vi "DestroyCommunication.vi"(8 "error in (no error)":errorcluster, 11 "Message Queues":T1) -> (0 "error out":errorcluster)   [LabVIEW 2017, in "Client.lvlib" / "CommsFrameWork.lvlib"]
doc: "Destroys all Queues and User Events."
uses:
  CommsFrameWork.lvlib
  TypeDefs/CommReferences.ctl
  ServerLib/SubLibs/Message Queue/MessageCluster.ctl
  ServerLib/SubLibs/Message Queue/Message Queue.lvlib
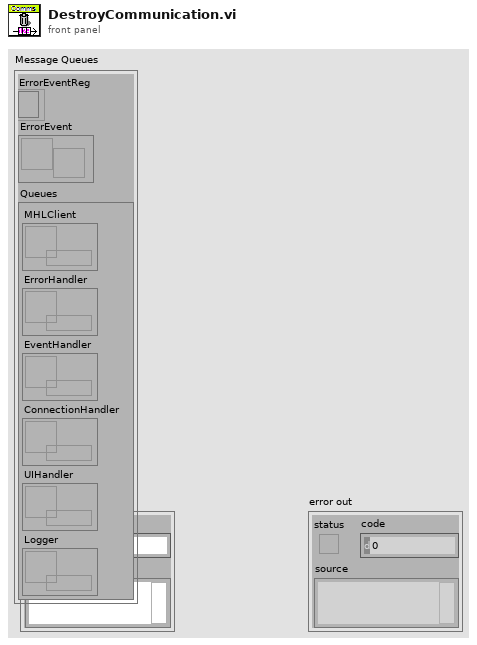
[diagram p1: front panel]
types:
  T1 = typedef "Client.lvlib/CommsFrameWork.lvlib/CommReferences.ctl" = cluster{"ErrorEventReg":refnum<event-registration>, "ErrorEvent":refnum<user-event>, "Queues":cluster{"MHLClient":refnum<queue>, "ErrorHandler":refnum<queue>, "EventHandler":refnum<queue>, "ConnectionHandler":refnum<queue>, "UIHandler":refnum<queue>, "Logger":refnum<queue>}}
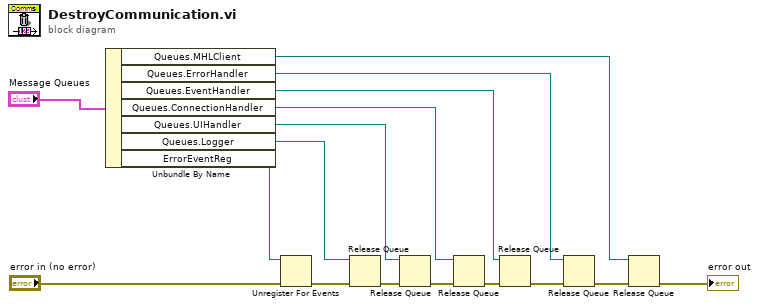
[diagram p0: block diagram]
diagram:
  n1 = Unbundle By Name("Message Queues") -> ("Queues.MHLClient"=w5:refnum<queue>, "Queues.ErrorHandler"=w6:refnum<queue>, "Queues.EventHandler"=w7:refnum<queue>, "Queues.ConnectionHandler"=w8:refnum<queue>, "Queues.UIHandler"=w9:refnum<queue>, "Queues.Logger"=w10:refnum<queue>, "ErrorEventReg"=w3:refnum<event-registration>)
  n2 = Unregister For Events(event registration refnum=w3, error in="error in (no error)") -> (error out=w1:errorcluster)
  n3 = Release Queue(queue=w10, error in (no error)=w1) -> (error out=w16:errorcluster)  [unwired: 1 in, 2 out]
  n4 = Release Queue(queue=w9, error in (no error)=w16) -> (error out=w15:errorcluster)  [unwired: 1 in, 2 out]
  n5 = Release Queue(queue=w8, error in (no error)=w15) -> (error out=w14:errorcluster)  [unwired: 1 in, 2 out]
  n6 = Release Queue(queue=w7, error in (no error)=w14) -> (error out=w13:errorcluster)  [unwired: 1 in, 2 out]
  n7 = Release Queue(queue=w6, error in (no error)=w13) -> (error out=w12:errorcluster)  [unwired: 1 in, 2 out]
  n8 = Release Queue(queue=w5, error in (no error)=w12) -> (error out=→"error out":errorcluster)  [unwired: 1 in, 2 out]
